vi "RandomHash.vi"() -> (3 "Numeric Control":u64)   [LabVIEW 2014]
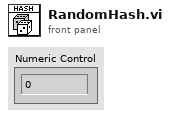
[diagram p1: front panel]
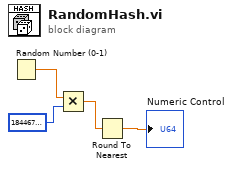
[diagram p0: block diagram]
diagram:
  n1 = Random Number (0-1)() -> (number: 0 to 1=w2:dbl)
  n2 = Multiply(x=w2, y=u64 18446744073709551615) -> (x*y=w4:dbl)
  n3 = Round To Nearest(number=w4) -> (nearest integer value=→"Numeric Control":dbl)
